vi "GObject Terminals.vi"(8 "error in (no error)":errorcluster, 11 "GObject in":refnum<vi>) -> (0 "error in (no error) (dup)":errorcluster, 1 "Class Name":string, 2 "Terms[]":refnum<vi>[](array[refnum]), 3 "Node Object":refnum<vi>, 4 "Tunnel Index":i32)   [LabVIEW 2020]
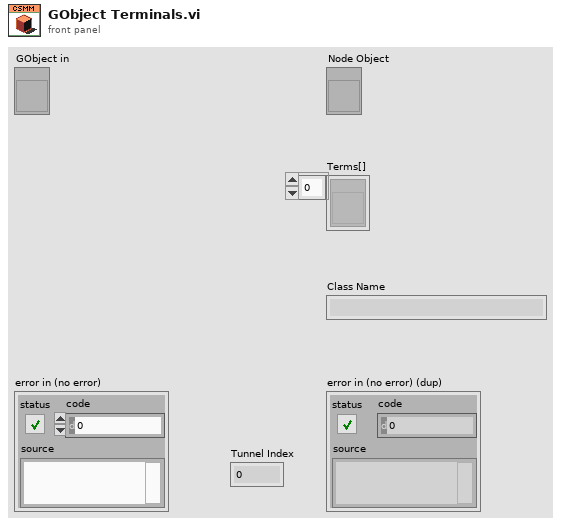
[diagram p1: front panel]
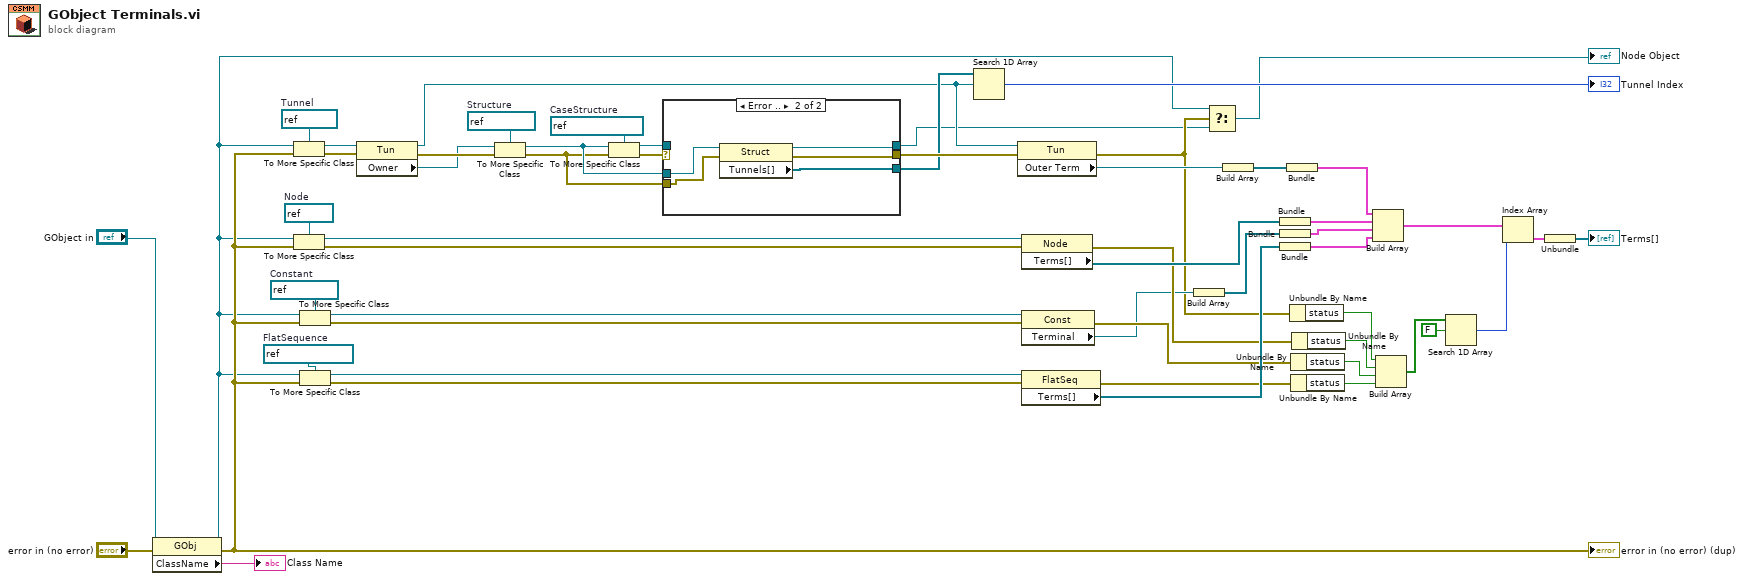
[diagram p0: block diagram]
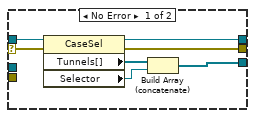
[diagram p2: hidden frame]
diagram:
  w5 = refnum<vi> refnum  # CaseStructure
  w14 = refnum<vi> refnum  # Structure
  w25 = refnum<vi> refnum  # Tunnel
  w38 = refnum<vi> refnum  # FlatSequence
  w35 = refnum<vi> refnum  # Constant
  w31 = refnum<vi> refnum  # Node
  n1 = property class="GObj"(reference="GObject in", error in="error in (no error)") -> (reference out=w7:refnum<vi>, error out=w19:errorcluster, "ClassName"=→"Class Name":string)
  "error in (no error) (dup)" <- w19
  n2 = To More Specific Class(target class=w25, reference=w7, error in=w19) -> (specific class reference=w18:refnum<vi>, error out=w17:errorcluster)
  n3 = To More Specific Class(target class=w31, reference=w7, error in=w19) -> (specific class reference=w30:refnum<vi>, error out=w29:errorcluster)
  n4 = To More Specific Class(target class=w35, reference=w7, error in=w19) -> (specific class reference=w33:refnum<vi>, error out=w32:errorcluster)
  n5 = To More Specific Class(target class=w38, reference=w7, error in=w19) -> (specific class reference=w39:refnum<vi>, error out=w40:errorcluster)
  n6 = property on="Property Node" class="Tun"(reference=w18, error in=w17) -> (reference out=w11:refnum<vi>, error out=w16:errorcluster, "Owner"=w15:refnum<vi>)
  n7 = To More Specific Class(target class=w14, reference=w15, error in=w16) -> (specific class reference=w2:refnum<vi>, error out=w1:errorcluster)
  n8 = To More Specific Class(target class=w5, reference=w2, error in=w1) -> (specific class reference=w3:refnum<vi>, error out=w4:errorcluster)
  n9 = case shown="Error .." w4 {
    selector: w4 -> [w59 _]
    tunnel: [w62 w66] -> w13
    tunnel: [w57 w63] -> w12
    tunnel: [w60 w64] -> w8
    tunnel: w3 -> [w58 _]
    tunnel: w2 -> [_ w67]
    tunnel: w1 -> [_ w65]
    frame No Error {
      n10 = property on="Property Node" class="CaseSel"(reference=w58, error in=w59) -> (reference out=w60:refnum<vi>, error out=w62:errorcluster, "Tunnels[]"=w61:refnum<vi>[], "Selector"=w56:refnum<vi>)
      n11 = Build Array (concatenate)(w61, w56) -> (w57:refnum<vi>[])
    }
    frame Error {
      n12 = property on="Property Node" class="Struct"(reference=w67, error in=w65) -> (reference out=w64:refnum<vi>, error out=w66:errorcluster, "Tunnels[]"=w63:refnum<vi>[])
    }
  }
  n13 = Search 1D Array(1D array=w12, element=w11) -> (index of element=→"Tunnel Index":i32)  [unwired: 1 in]
  n14 = property on="Property Node" class="Tun"(reference=w11, error in=w13) -> (error out=w9:errorcluster, "Outer Term"=w24:refnum<vi>)  [unwired: 1 out]
  n15 = property on="Property Node" class="Node"(reference=w30, error in=w29) -> (error out=w36:errorcluster, "Terms[]"=w47:refnum<vi>[])  [unwired: 1 out]
  n16 = property on="Property Node" class="Const"(reference=w33, error in=w32) -> (error out=w37:errorcluster, "Terminal"=w34:refnum<vi>)  [unwired: 1 out]
  n17 = property on="Property Node" class="FlatSeq"(reference=w39, error in=w40) -> (error out=w41:errorcluster, "Terms[]"=w49:refnum<vi>[])  [unwired: 1 out]
  n18 = Build Array(w34) -> (w48:refnum<vi>[])
  n19 = Select(t=w7, s=w9, f=w8) -> (s? t:f=→"Node Object":refnum<vi>)
  n20 = Build Array(w24) -> (w23:refnum<vi>[])
  n21 = Bundle("Terms[]"=w47) -> (w22:cluster{"Terms[]":refnum<vi>[]})  [unwired: 1 in]
  n22 = Bundle(w48) -> (w50:cluster{refnum<vi>[]})  [unwired: 1 in]
  n23 = Bundle("Terms[]"=w49) -> (w51:cluster{"Terms[]":refnum<vi>[]})  [unwired: 1 in]
  n24 = Bundle(w23) -> (w21:cluster{refnum<vi>[]})  [unwired: 1 in]
  n25 = Unbundle By Name(w9) -> ("status"=w20:bool)
  n26 = Unbundle By Name(w37) -> ("status"=w43:bool)
  n27 = Unbundle By Name(w41) -> ("status"=w44:bool)
  n28 = Unbundle By Name(w36) -> ("status"=w42:bool)
  n29 = Build Array(w21, w22, w50, w51) -> (w52:cluster{"Terms[]":refnum<vi>[]}[])
  n30 = Build Array(w20, w42, w43, w44) -> (w45:bool[])
  n31 = Search 1D Array(1D array=w45, element=FALSE) -> (index of element=w53:i32)  [unwired: 1 in]
  n32 = Index Array(array=w52, index=w53) -> (element=w54:cluster{"Terms[]":refnum<vi>[]})
  n33 = Unbundle(w54) -> ("Terms[]"=→"Terms[]":refnum<vi>[])
